vi "3D-Flat_4to sraightness.vi"(9 "Z":dbl[](array[numeric]), 10 "Y":dbl[](array[numeric]), 11 "X":dbl[](array[numeric])) -> (0 "x-y":dbl, 1 "C":dbl, 2 "B":dbl, 3 "A":dbl, 5 "£GZ":dbl[](array[numeric]))   [LabVIEW 2015]
uses:
  <vilib>/Analysis/7linalg.llb/Solve Linear Equations (single right hand).vi
  <vilib>/Analysis/baseanly.llb/Solve Linear Equations By Cholesky.vi
  <vilib>/Analysis/baseanly.llb/Real Matrix to Compact Array.vi
  <vilib>/Analysis/baseanly.llb/Real Compact Tri-Matrix Linear Eqs.vi
  <vilib>/Analysis/7linalg.llb/Solve Linear Eqs (General).vi
  <vilib>/Analysis/7linalg.llb/Solve Linear Eqs (Gen, single right hand).vi
  <vilib>/Analysis/NI_AALPro.lvlib
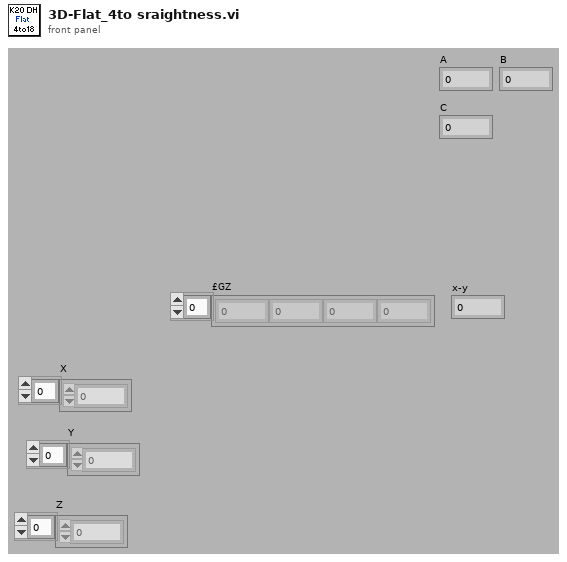
[diagram p1: front panel]
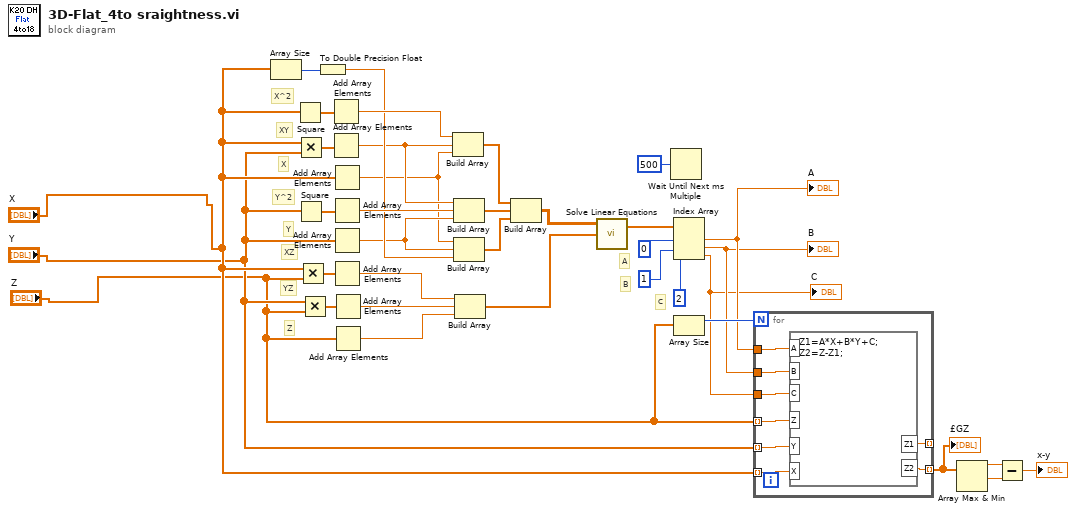
[diagram p0: block diagram]
diagram:
  # "C"
  # "B"
  # "A"
  # "Z"
  # "XZ"
  # "YZ"
  # "Y"
  # "Y^2"
  # "XY"
  # "X"
  # "X^2"
  n1 = Array Size(array="X") -> (size(s)=w25:i32)
  n2 = Square(x="X") -> (x^2=w36:dbl[])
  n3 = Multiply(x="X", y="Y") -> (x*y=w9:dbl[])
  n4 = Square(x="Y") -> (x^2=w35:dbl[])
  n5 = Multiply(x="X", y="Z") -> (x*y=w34:dbl[])
  n6 = Multiply(x="Y", y="Z") -> (x*y=w33:dbl[])
  n7 = To Double Precision Float(number=w25) -> (double precision float=w24:dbl)
  n8 = Add Array Elements(numeric array=w36) -> (sum=w32:dbl)
  n9 = Add Array Elements(numeric array=w9) -> (sum=w8:dbl)
  n10 = Add Array Elements(numeric array="X") -> (sum=w7:dbl)
  n11 = Add Array Elements(numeric array=w35) -> (sum=w31:dbl)
  n12 = Add Array Elements(numeric array="Y") -> (sum=w20:dbl)
  n13 = Add Array Elements(numeric array=w34) -> (sum=w30:dbl)
  n14 = Add Array Elements(numeric array=w33) -> (sum=w29:dbl)
  n15 = Add Array Elements(numeric array="Z") -> (sum=w19:dbl)
  n16 = Build Array(w32, w8, w7) -> (w28:dbl[])
  n17 = Build Array(w8, w31, w20) -> (w27:dbl[])
  n18 = Build Array(w7, w20, w24) -> (w26:dbl[])
  n19 = Build Array(w30, w29, w19) -> (w5:dbl[])
  n20 = Build Array(w28, w27, w26) -> (w6:dbl[][])
  n21 = call-poly <vilib>:"Solve Linear Equations.vi"("Known Vector"=w5, "Input Matrix"=w6) -> ("Solution Vector"=w13:dbl[])  [unwired: 1 in, 1 out]
  n22 = Wait Until Next ms Multiple(millisecond multiple=u32 500) -> ()  [unwired: 1 out]
  n23 = Index Array(array=w13, index #1=0 ("index"), index #2=1 ("index"), index #3=2 ("index")) -> (element #1=w12:dbl, element #2=w11:dbl, element #3=w10:dbl)
  "A" <- w12
  "B" <- w11
  "C" <- w10
  n24 = Array Size(array="Z") -> (size(s)=w17:i32)
  n25 = for {
    N: w17 -> [_]
    tunnel: "X" -> [w44] mode=indexing
    tunnel: "Y" -> [w43] mode=indexing
    tunnel: "Z" -> [w42] mode=indexing
    tunnel: w10 -> [w41]
    tunnel: w11 -> [w40]
    tunnel: w12 -> [w39]
    tunnel: [w38] -> w1 mode=indexing
    tunnel: [w37] -> _ mode=indexing
    n26 = formula code="Z1=A*X+B*Y+C;\nZ2=Z-Z1;"("Z"=w42, "Y"=w43, "X"=w44, "A"=w39, "B"=w40, "C"=w41) -> ("Z2"=w38:dbl, "Z1"=w37:dbl)
  }
  "£GZ" <- w1
  n27 = Array Max & Min(array=w1) -> (max value=w16:dbl, min value=w15:dbl)  [unwired: 2 out]
  n28 = Subtract(x=w16, y=w15) -> (x-y=→"x-y":dbl)
